vi "Check for Valid Test Number.vi"(0 "Session Handle in":T1, 7 "element":i64, 11 "error in (no error)":errorcluster) -> (4 "Session Handle out":T1, 8 "Valid Test Number?":bool, 15 "error out":errorcluster)   [LabVIEW 2018, in "Test Number and Bin Generator.lvlib" / "Test Number and Bin Generator.lvclass"]
uses:
  Test Number and Bin Generator.lvclass
  Typedefs/Session Handle.ctl
  Test Number and Bin Generator.lvclass/Test Number and Bin Generator.ctl
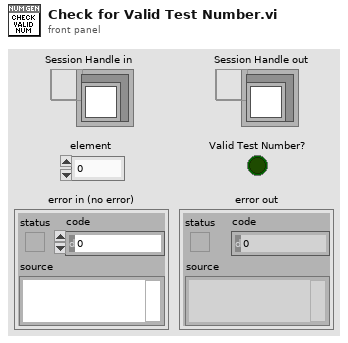
[diagram p1: front panel]
types:
  T1 = typedef "Test Number and Bin Generator.lvlib/Test Number and Bin Generator.lvclass/Session Handle.ctl" = refnum<data-value>
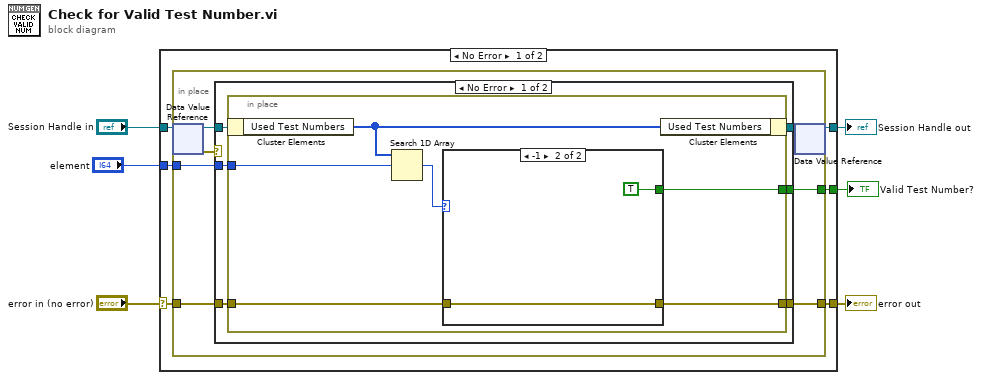
[diagram p0: block diagram]
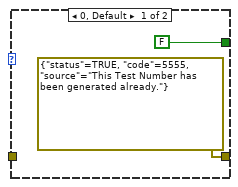
[diagram p2: hidden frame]
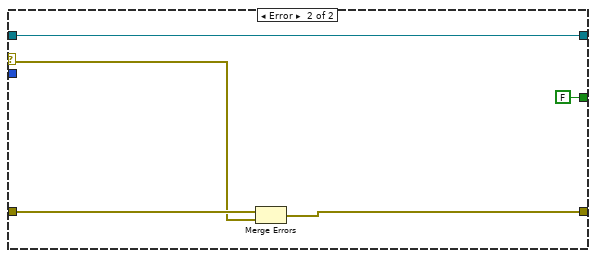
[diagram p3: hidden frame]
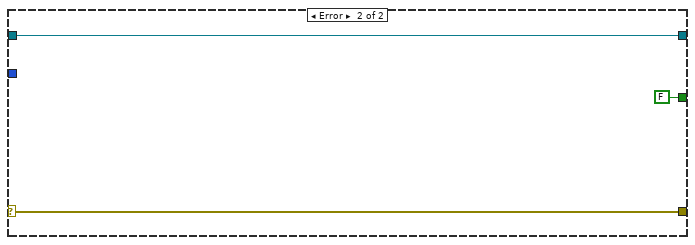
[diagram p4: hidden frame]
diagram:
  n1 = case shown="No Error" "error in (no error)" {
    selector: "error in (no error)" -> [w10 w42]
    tunnel: "Session Handle in" -> [w12 w43]
    tunnel: [w11 w43] -> w5
    tunnel: [w9 w42] -> w4
    tunnel: "element" -> [w8 _]
    tunnel: [w7 FALSE] -> w1
    frame No Error {
      n2 = in-place {
        in-place-border: w10 -> [w15]
        in-place-border: [w18] -> w9
        in-place-border: w8 -> [w14]
        in-place-border: [w13] -> w7
        n3 = in-place-dvr #1(w12) -> (w19:refnum<class "Test Number and Bin Generator.lvclass">, w16:errorcluster)
        n4 = case shown="No Error" w16 {
          selector: w16 -> [_ w39]
          tunnel: w19 -> [w25 w37]
          tunnel: [w24 w38] -> w18
          tunnel: [w23 w37] -> w17
          tunnel: w15 -> [w22 w40]
          tunnel: w14 -> [w21 _]
          tunnel: [w20 FALSE] -> w13
          frame No Error {
            n5 = in-place {
              in-place-border: [w27] -> w24
              in-place-border: w22 -> [w28]
              in-place-border: w21 -> [w30]
              in-place-border: [w26] -> w20
              n6 = in-place-cluster #2(w25) -> ("Used Test Numbers"=w31:i64[])
              n7 = Search 1D Array(1D array=w31, element=w30) -> (index of element=w29:i32)  [unwired: 1 in]
              n8 = case shown="-1" w29 {
                tunnel: w28 -> [_ w35]
                tunnel: [errorcluster {"status"=TRUE, "code"=5555, "source"="This Test Number has been generated already."} ("error IO") w35] -> w27
                tunnel: [FALSE TRUE] -> w26
                frame 0, Default {
                }
                frame -1 {
                }
              }
              n9 = in-place-cluster #2("Used Test Numbers"=w31) -> (w23:refnum<class "Test Number and Bin Generator.lvclass">)
            }
          }
          frame Error {
            n10 = Merge Errors(w40, w39) -> (w38:errorcluster)
          }
        }
        n11 = in-place-dvr #1(w17) -> (w11:T1)  [unwired: 1 out]
      }
    }
    frame Error {
    }
  }
  "Session Handle out" <- w5
  "error out" <- w4
  "Valid Test Number?" <- w1
